vi "Merge Sort Record Entries.vi"(0 "Sorted Entries A":string[](array[string]), 1 "Ignore Duplicates? (F)":bool, 3 "Sorted Entries B":string[](array[string])) -> (6 "Sorted Entries":string[](array[string]))   [LabVIEW 2013, in "Data Log Fetcher.lvlib"]
uses:
  Data Log Fetcher.lvlib
panel:
  out "A Index":i32
  out "B Index":i32
  out "B Count":i32
  out "A Count":i32
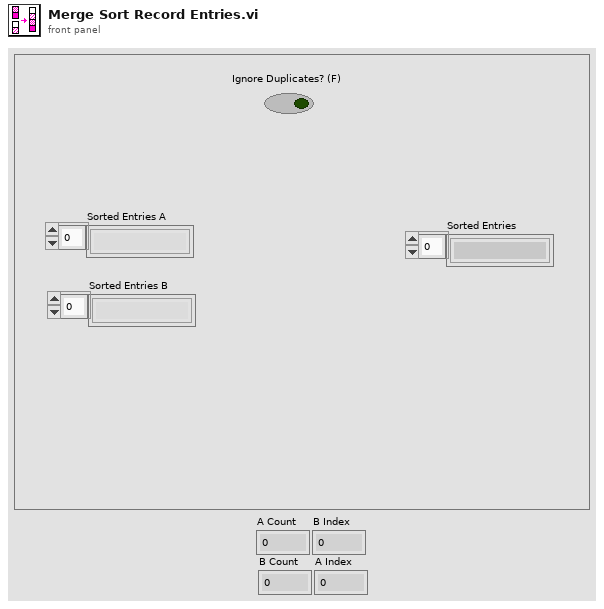
[diagram p1: front panel]
types:
  T1 = enum16{"JAN", "FEB", "MAR", "APR", "MAY", "JUN", "JUL", "AUG", "SEP", "OCT", "NOV", "DEC"}
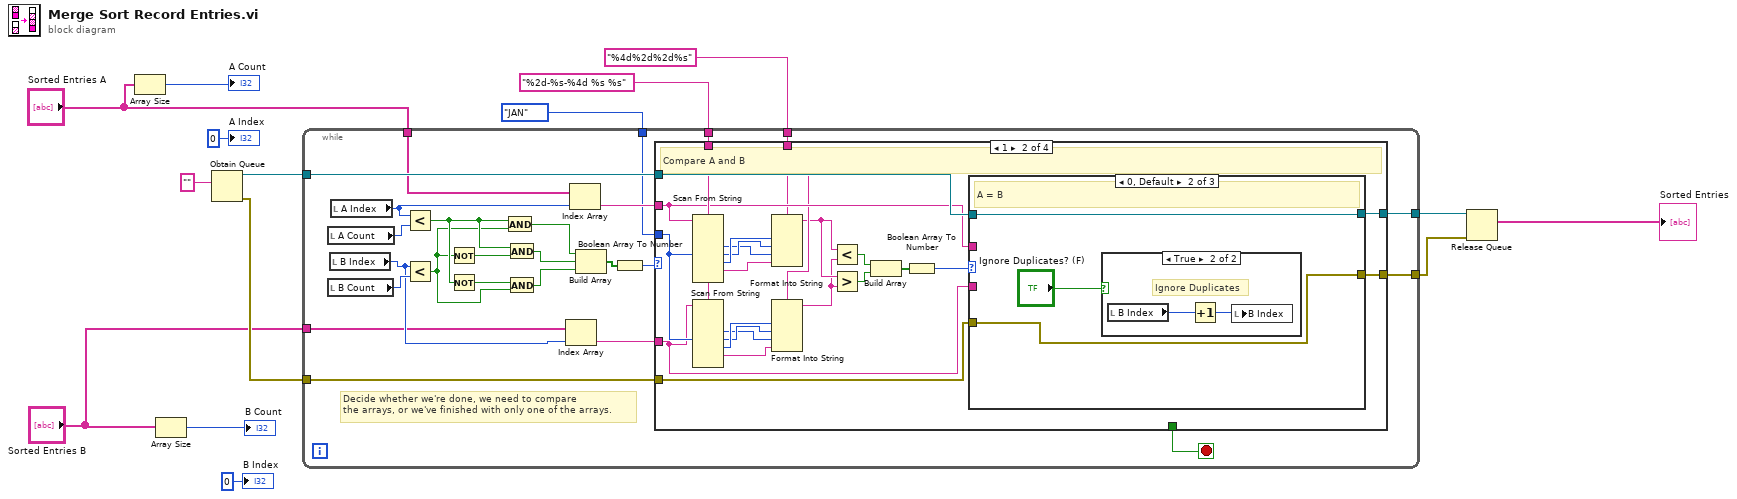
[diagram p0: block diagram]
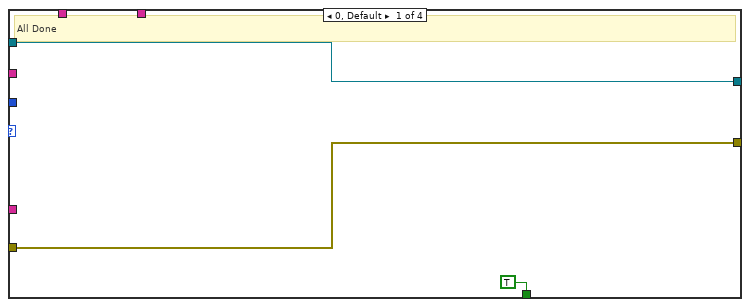
[diagram p2: hidden frame]
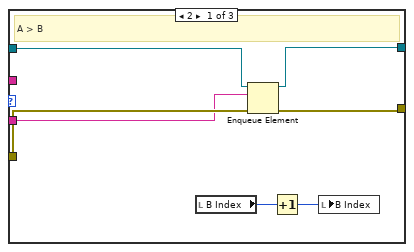
[diagram p3: hidden frame]
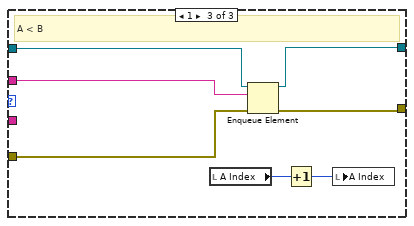
[diagram p5: hidden frame]
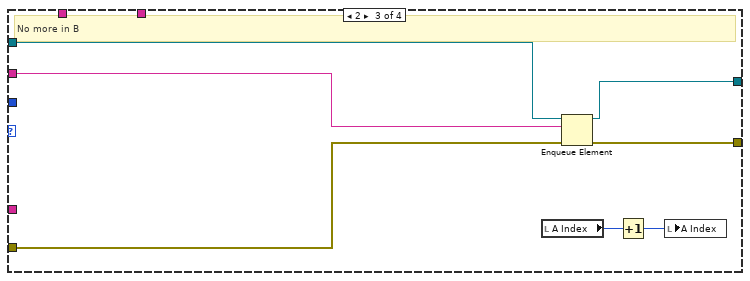
[diagram p6: hidden frame]
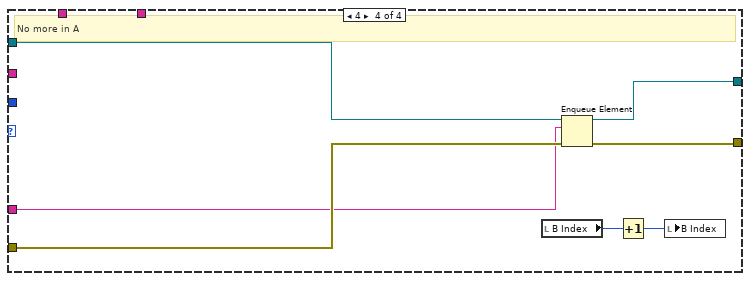
[diagram p7: hidden frame]
diagram:
  n1 = Array Size(array="Sorted Entries A") -> (size(s)=→"A Count":i32)
  n2 = Array Size(array="Sorted Entries B") -> (size(s)=→"B Count":i32)
  n3 = Obtain Queue(element data type="") -> (queue out=w14:refnum<queue>, error out=w13:errorcluster)  [unwired: 4 in, 1 out]
  n4 = while {
    tunnel: w14 -> [w29]
    tunnel: [w28] -> w10
    tunnel: [w27] -> w15
    tunnel: w13 -> [w26]
    tunnel: "Sorted Entries A" -> [w20]
    tunnel: "Sorted Entries B" -> [w19]
    tunnel: "%2d-%s-%4d %s %s" ("format string") -> [w18]
    tunnel: "%4d%2d%2d%s" ("format string") -> [w17]
    tunnel: T1."JAN" ("Months") -> [w16]
    stop <- w21 stop-if-true
    # "Decide whether we're done, we need to compare\nthe arrays, or we've finished with only one of the arrays."
    n5 = local read "A Count"() -> (w40:i32)
    n6 = local read "B Count"() -> (w39:i32)
    n7 = local read "B Index"() -> (w24:i32)
    n8 = local read "A Index"() -> (w25:i32)
    n9 = Less?(x=w25, y=w40) -> (x < y?=w36:bool)
    n10 = Less?(x=w24, y=w39) -> (x < y?=w35:bool)
    n11 = Not(x=w35) -> (.not. x?=w33:bool)
    n12 = Not(x=w36) -> (.not. x?=w32:bool)
    n13 = And(x=w36, y=w35) -> (x .and. y?=w38:bool)
    n14 = And(x=w36, y=w33) -> (x .and. y?=w37:bool)
    n15 = And(x=w32, y=w35) -> (x .and. y?=w34:bool)
    n16 = Index Array(array=w19, index=w24) -> (element=w23:string)
    n17 = Index Array(array=w20, index=w25) -> (element=w22:string)
    n18 = Build Array(w38, w37, w34) -> (w31:bool[])
    n19 = Boolean Array To Number(Boolean array=w31) -> (number=w30:u32)
    n20 = case shown="1" w30 {
      tunnel: w29 -> [w43 w66 w92 w99]
      tunnel: w22 -> [_ w53 w90 _]
      tunnel: w23 -> [_ w52 _ w97]
      tunnel: w26 -> [w42 w63 w91 w98]
      tunnel: [w42 w65 w88 w95] -> w28
      tunnel: [w43 w64 w89 w96] -> w27
      tunnel: [TRUE _ _ _] -> w21
      tunnel: w18 -> [_ w55 _ _]
      tunnel: w17 -> [_ w51 _ _]
      tunnel: w16 -> [_ w54 _ _]
      frame 0, Default {
        # "All Done"
      }
      frame 1 {
        # "Compare A and B"
        n21 = Scan From String(format string=w55, input string=w53, default 2=w54) -> (output 1=w60:i32, output 2=w61:T1, output 3=w62:i32, output 4=w59:string)  [unwired: 7 in, 3 out]
        n22 = Scan From String(format string=w55, input string=w52, default 2=w54) -> (output 1=w56:i32, output 2=w57:T1, output 3=w58:i32, output 4=w50:string)  [unwired: 7 in, 3 out]
        n23 = Format Into String(format string=w51, w62, w61, w60, w59) -> (resulting string=w46:string)  [unwired: 2 in, 1 out]
        n24 = Format Into String(format string=w51, w58, w57, w56, w50) -> (resulting string=w45:string)  [unwired: 2 in, 1 out]
        n25 = Less?(x=w46, y=w45) -> (x < y?=w47:bool)
        n26 = Greater?(x=w46, y=w45) -> (0:w48:bool)
        n27 = Build Array(w47, w48) -> (w49:bool[])
        n28 = Boolean Array To Number(Boolean array=w49) -> (number=w44:u32)
        n29 = case shown="0, Default" w44 {
          tunnel: w66 -> [w73 w74 w85]
          tunnel: w53 -> [_ _ w84]
          tunnel: w52 -> [w67 _ _]
          tunnel: w63 -> [w72 w75 w83]
          tunnel: [w70 w75 w81] -> w65
          tunnel: [w71 w74 w82] -> w64
          frame 2 {
            # "A > B"
            n30 = local read "B Index"() -> (w68:i32)
            n31 = Enqueue Element(queue=w73, element=w67, error in (no error)=w72) -> (queue out=w71:refnum<queue>, error out=w70:errorcluster)  [unwired: 1 in, 1 out]
            n32 = Increment(x=w68) -> (x+1=w69:i32)
            n33 = local write "B Index"(w69) -> ()
          }
          frame 0, Default {
            # "A = B"
            n34 = case shown="True" "Ignore Duplicates? (F)" {
              frame False {
              }
              frame True {
                # "Ignore Duplicates"
                n35 = local read "B Index"() -> (w78:i32)
                n36 = Increment(x=w78) -> (x+1=w77:i32)
                n37 = local write "B Index"(w77) -> ()
              }
            }
          }
          frame 1 {
            # "A < B"
            n38 = local read "A Index"() -> (w79:i32)
            n39 = Enqueue Element(queue=w85, element=w84, error in (no error)=w83) -> (queue out=w82:refnum<queue>, error out=w81:errorcluster)  [unwired: 1 in, 1 out]
            n40 = Increment(x=w79) -> (x+1=w80:i32)
            n41 = local write "A Index"(w80) -> ()
          }
        }
      }
      frame 2 {
        # "No more in B"
        n42 = local read "A Index"() -> (w86:i32)
        n43 = Enqueue Element(queue=w92, element=w90, error in (no error)=w91) -> (queue out=w89:refnum<queue>, error out=w88:errorcluster)  [unwired: 1 in, 1 out]
        n44 = Increment(x=w86) -> (x+1=w87:i32)
        n45 = local write "A Index"(w87) -> ()
      }
      frame 4 {
        # "No more in A"
        n46 = local read "B Index"() -> (w93:i32)
        n47 = Enqueue Element(queue=w99, element=w97, error in (no error)=w98) -> (queue out=w96:refnum<queue>, error out=w95:errorcluster)  [unwired: 1 in, 1 out]
        n48 = Increment(x=w93) -> (x+1=w94:i32)
        n49 = local write "B Index"(w94) -> ()
      }
    }
  }
  n50 = Release Queue(queue=w15, error in (no error)=w10) -> (remaining elements=→"Sorted Entries":string[])  [unwired: 1 in, 2 out]
  "A Index" <- 0 ("A Index")
  "B Index" <- 0 ("B Index")
